vi "Create Dataset 2D Integer.vi"(7 "Chunk size":u64, 8 "error in (no error)":errorcluster, 9 "Datatype":u64[][](array[numeric]), 10 "Dataset name":string, 11 "Location id in":i32) -> (0 "error out":errorcluster, 3 "Dataset id":i32)   [LabVIEW 2011]
uses:
  Release/HDF5Tools.dll
  HDF5Tools.lvlib
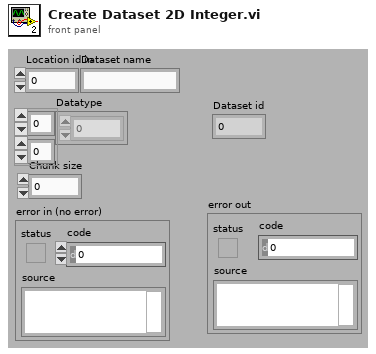
[diagram p1: front panel]
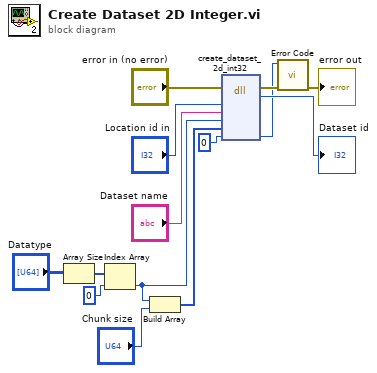
[diagram p0: block diagram]
diagram:
  n1 = Array Size(array="Datatype") -> (size(s)=w10:i32[])
  n2 = Index Array(array=w10, index=0) -> (element=w4:i32)
  n3 = Build Array(w4, "Chunk size") -> (w5:u64[])
  n4 = dll-call lib="F:/HDF5Tools/Release/HDF5Tools.dll" fn="create_dataset_2d_int32"(error in="error in (no error)", "loc_id"="Location id in", "name"="Dataset name", "dim1"=w4, "chunks"=w5, "error"=0) -> (error out=w2:errorcluster, "dataset_id"=→"Dataset id":i32, "error"=w1:i32)  [unwired: 6 in, 1 out]
  n5 = call "Error Code.vi"("Error in"=w2, "Error code"=w1) -> ("Error out"=→"error out":errorcluster)  [unwired: 9 in]
